vi "Drone Face Recognition.vi"() -> ()   [LabVIEW 2014]
doc: "This example shows how to use the Lucas Kanade Pyramid motion estimation VI to track features in a sequence of images in NI Vision. The VI reads the frames from an AVI file and tracks user specified features in the image from frame to frame."
uses:
  <vilib>/vision/NI_Vision_Development_Module.lvlib
panel:
  out "DroneGetVideoError":errorcluster
  out "Face Found":bool
  in  "Show Templates":bool=TRUE
  out "Preview":T1(plugin-control)
  in  "Lip Min Score":sgl=700.0
  in  "Nose Min Score":sgl=700.0
  in  "Eye Min Score":sgl=700.0
  out "Lips Template":T1(plugin-control)
  out "Nose Template":T1(plugin-control)
  out "Eye Template":T1(plugin-control)
  in  "Options":T2={"Level"=4, "maxiteration"=20, "windowsize"=20, "threshold"=1.0}
  in  "Stop":bool
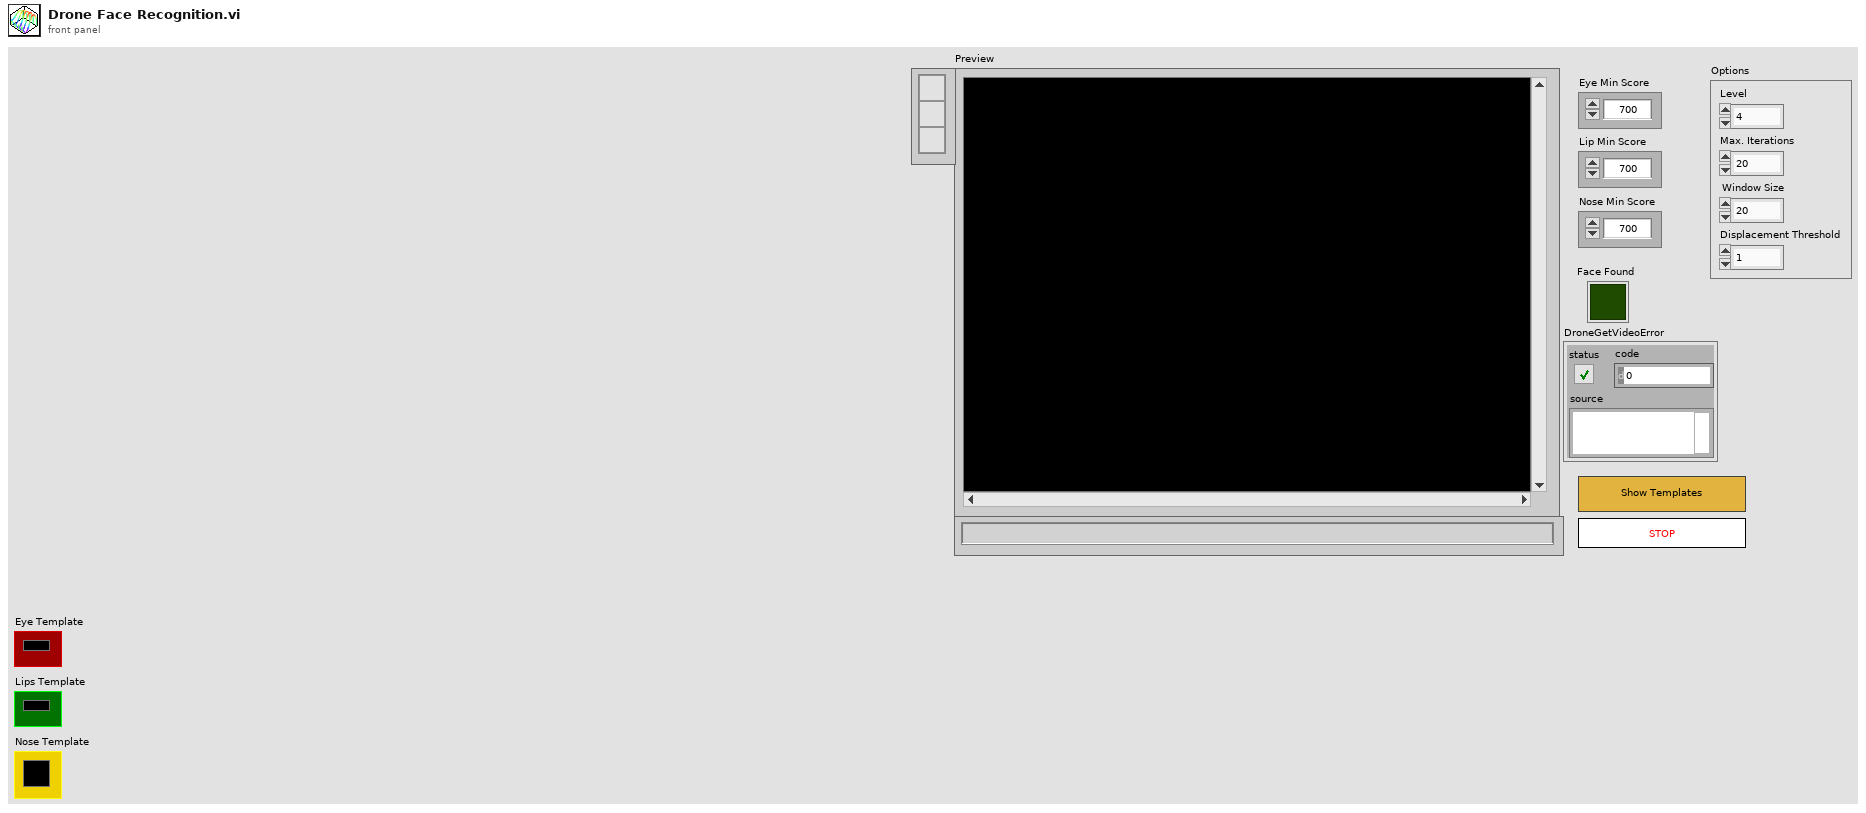
[diagram p1: front panel]
types:
  T1 = typedef "IMAQ Image.ctl" = refnum<image>
  T2 = cluster{"Level":i32, "maxiteration":i32, "windowsize":i32, "threshold":dbl}
  T3 = typedef "Image Type" = u32
  T4 = cluster{"Position":cluster{"x":sgl, "y":sgl}, "Angle":sgl, "Scale":sgl, "Score":sgl, "Bounding Box":cluster{"x":sgl, "y":sgl}[]}[]
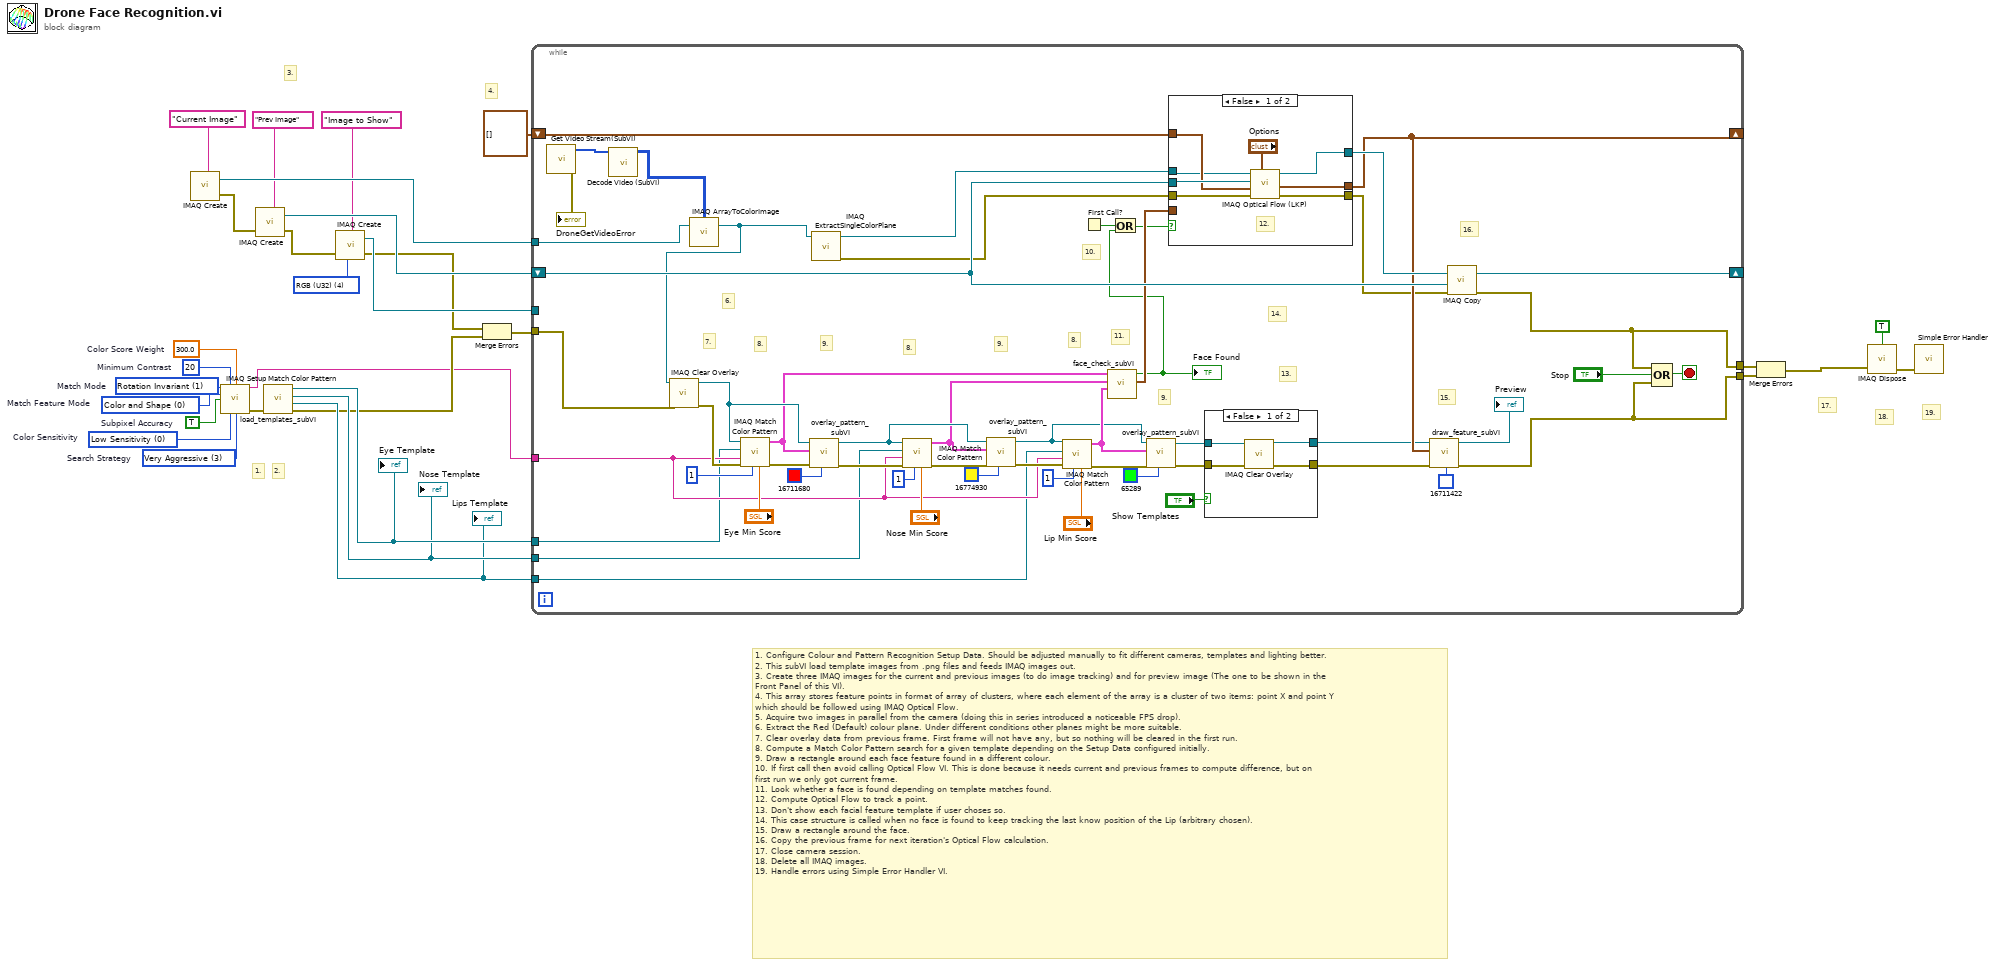
[diagram p0: block diagram]
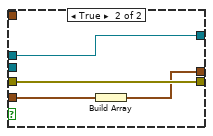
[diagram p3: hidden frame]
diagram:
  w15 = T3 4 items=["Grayscale (U8)", "Grayscale (I16)", "Grayscale (SGL)", "Complex (CSG)", "RGB (U32)", "HSL (U32)", "RGB (U64)", "Grayscale (U16)"] ("Image Type")
  w19 = TRUE  # Subpixel Accuracy
  w25 = u32 0 items=["Color and Shape", "Color", "Shape"]  # Match Feature Mode
  w24 = u32 3 items=["Conservative", "Balance", "Aggressive", "Very Aggressive"]  # Search Strategy
  w23 = 20  # Minimum Contrast
  w22 = sgl 300.0  # Color Score Weight
  w21 = u32 0 items=["Low Sensitivity", "Medium Sensitivity", "High Sensitivity"]  # Color Sensitivity
  w20 = u32 1 items=["Shift Invariant", "Rotation Invariant"]  # Match Mode
  # "1. Configure Colour and Pattern Recognition Setup Data. Should be adjusted manually to fit different cameras, templates and lighting better.\n2. This subVI load template images from .png files and feeds IMAQ images out.\n3. Create three IMAQ images for the current and previous images (to do image tracking) and for preview image (The one to be shown in the\nFront Panel of this VI).\n4. This array stores feature points in format of array of clusters, where each element of the array is a cluster of two items: point X and point Y \nwhich should be followed using IMAQ Optical Flow.\n5. Acquire two images in parallel from the camera (doing this in series introduced a noticeable FPS drop).\n6. Extract the Red (Default) colour plane. Under different conditions other planes might be more suitable.\n7. Clear overlay data from previous frame. First frame will not have any, but so nothing will be cleared in the first run.\n8. Compute a Match Color Pattern search for a given template depending on the Setup Data configured initially.\n9. Draw a rectangle around each face feature found in a different colour.\n10. If first call then avoid calling Optical Flow VI. This is done because it needs current and previous frames to compute difference, but on\nfirst run we only got current frame.\n11. Look whether a face is found depending on template matches found.\n12. Compute Optical Flow to track a point.\n13. Don't show each facial feature template if user choses so.\n14. This case structure is called when no face is found to keep tracking the last know position of the Lip (arbitrary chosen).\n15. Draw a rectangle around the face.\n16. Copy the previous frame for next iteration's Optical Flow calculation.\n17. Close camera session.\n18. Delete all IMAQ images.\n19. Handle errors using Simple Error Handler VI."
  # "19."
  # "17."
  # "4."
  # "3."
  # "3."
  # "3."
  # "2."
  # "1."
  # "18."
  n1 = call "IMAQ Create"("Image Name"="Current Image") -> ("New Image"=w29:T1, "error out"=w9:errorcluster)  [unwired: 3 in, 1 out]
  n2 = call "IMAQ Setup Match Color Pattern"("Match Mode"=w20, "Minimum Contrast"=w23, "Color Score Weight"=w22, "Match Feature Mode"=w25, "Subpixel Accuracy"=w19, "Color Sensitivity"=w21, "Search Strategy"=w24) -> ("Match Color Pattern Setup Data"=w4:string, "error out"=w18:errorcluster)  [unwired: 7 in]
  n3 = call "IMAQ Create"("Image Name"="Prev Image", "error in (no error)"=w9) -> ("New Image"=w26:T1, "error out"=w8:errorcluster)  [unwired: 2 in, 1 out]
  n4 = call "load_templates_subVI.vi"("error in (no error)"=w18) -> ("error out"=w6:errorcluster, "Lips Template"=w12:T1, "Nose Template"=w13:T1, "Eye Template"=w14:T1)  [unwired: 7 in]
  "Eye Template" <- w14
  "Nose Template" <- w13
  "Lips Template" <- w12
  n5 = call "IMAQ Create"("Image Name"="Image to Show", "Image Type"=w15, "error in (no error)"=w8) -> ("New Image"=w16:T1, "error out"=w7:errorcluster)  [unwired: 1 in, 1 out]
  n6 = Merge Errors(w7, w6) -> (w5:errorcluster)
  n7 = while {
    tunnel: w29 -> [w34]
    shift-right: [w83] -> _
    shift-left: w26 -> [w84]
    shift-right: [w51] -> _
    shift-left: cluster{"X":sgl, "Y":sgl}[] [] ("Feature Points Out") -> [w82]
    tunnel: w4 -> [w57]
    tunnel: w14 -> [w56]
    tunnel: w13 -> [w55]
    tunnel: w12 -> [w54]
    tunnel: w16 -> [_]
    tunnel: w5 -> [w36]
    tunnel: [w41] -> w3
    tunnel: [w40] -> w2
    stop <- w43 stop-if-true
    # "10."
    # "16."
    # "15."
    # "14."
    # "13."
    # "11."
    # "9."
    # "8."
    # "9."
    # "8."
    # "9."
    # "8."
    # "7."
    # "6."
    n8 = call "Get Video Stream(SubVI).vi"() -> ("error out"=→"DroneGetVideoError":errorcluster, "ImgData"=w35:u8[])  [unwired: 10 in]
    n9 = call "Decode Video (SubVI).vi"("ImgData"=w35) -> ("Array"=w32:u32[][])  [unwired: 9 in, 1 out]
    n10 = call "IMAQ ArrayToColorImage"("Image Pixels (U32)"=w32, "Image"=w34) -> ("Image Out"=w31:T1)  [unwired: 3 in, 1 out]
    n11 = call "IMAQ Clear Overlay"("error in (no error)"=w36, "Image"=w31) -> ("error out"=w78:errorcluster, "Image Out"=w64:T1)  [unwired: 8 in]
    n12 = call "IMAQ Match Color Pattern"("Minimum Match Score"="Eye Min Score", "Number of Matches Requested"=1, "error in (no error)"=w78, "Match Color Pattern Setup Data"=w57, "Template Image"=w56, "Image"=w64) -> ("error out"=w77:errorcluster, "Matches"=w61:T4)  [unwired: 3 in, 1 out]
    n13 = call "overlay_pattern_subVI.vi"("Color"=u32 16711680, "error in"=w77, "Matches"=w61, "Image"=w64) -> ("error out"=w74:errorcluster, "Image Out"=w71:T1)  [unwired: 6 in]
    n14 = call "IMAQ ExtractSingleColorPlane"("Image Src"=w31) -> ("error out"=w81:errorcluster, "Image Dst Out"=w80:T1)  [unwired: 9 in]
    n15 = call "IMAQ Match Color Pattern"("Minimum Match Score"="Nose Min Score", "Number of Matches Requested"=1, "error in (no error)"=w74, "Match Color Pattern Setup Data"=w57, "Template Image"=w55, "Image"=w71) -> ("error out"=w72:errorcluster, "Matches"=w60:T4)  [unwired: 3 in, 1 out]
    n16 = call "overlay_pattern_subVI.vi"("Color"=u32 16774930, "error in"=w72, "Matches"=w60, "Image"=w71) -> ("error out"=w70:errorcluster, "Image Out"=w58:T1)  [unwired: 6 in]
    n17 = call "IMAQ Match Color Pattern"("Minimum Match Score"="Lip Min Score", "Number of Matches Requested"=1, "error in (no error)"=w70, "Match Color Pattern Setup Data"=w57, "Template Image"=w54, "Image"=w58) -> ("error out"=w69:errorcluster, "Matches"=w59:T4)  [unwired: 3 in, 1 out]
    n18 = First Call?() -> (First Call?: T/F=w37:bool)
    n19 = call "face_check_subVI.vi"("Lips Match"=w59, "Nose Match"=w60, "Eye Match"=w61) -> ("Lip Position"=w53:cluster{"x":sgl, "y":sgl}, "Face Found"=w39:bool)  [unwired: 6 in, 1 out]
    "Face Found" <- w39
    n20 = Or(x=w37, y=w39) -> (x .or. y?=w38:bool)
    n21 = call "overlay_pattern_subVI.vi"("Color"=u32 65289, "error in"=w69, "Matches"=w59, "Image"=w58) -> ("error out"=w47:errorcluster, "Image Out"=w49:T1)  [unwired: 6 in]
    n22 = case shown="False" w38 {
      tunnel: w84 -> [w98 _]
      tunnel: w82 -> [w97 _]
      tunnel: [w96 w99] -> w51
      tunnel: w81 -> [w95 w102]
      tunnel: w80 -> [w91 w101]
      tunnel: [w93 w101] -> w79
      tunnel: [w92 w102] -> w44
      tunnel: w53 -> [_ w100]
      frame False {
        # "12."
        n23 = call "IMAQ Optical Flow (LKP)"("Options"="Options", "error in (no error)"=w95, "Feature Points In"=w97, "Previous Frame"=w98, "Current Frame"=w91) -> ("error out"=w92:errorcluster, "Feature Points Out"=w96:cluster{"X":sgl, "Y":sgl}[], "Current Frame Out (dup)"=w93:T1)  [unwired: 1 in, 3 out]
      }
      frame True {
        n24 = Build Array(w100) -> (w99:cluster{"x":sgl, "y":sgl}[])
      }
    }
    n25 = case shown="False" "Show Templates" {
      tunnel: w49 -> [w88 w90]
      tunnel: [w87 w90] -> w48
      tunnel: w47 -> [w86 w89]
      tunnel: [w85 w89] -> w45
      frame False {
        n26 = call "IMAQ Clear Overlay"("error in (no error)"=w86, "Image"=w88) -> ("error out"=w85:errorcluster, "Image Out"=w87:T1)  [unwired: 8 in]
      }
      frame True {
      }
    }
    n27 = call "draw_feature_subVI.vi"("Color"=u32 16711422, "Error In"=w45, "Feature Ponts"=w51, "Image"=w48) -> ("Error Out"=w40:errorcluster, "Image Out"=→"Preview":T1)  [unwired: 6 out]
    n28 = call "IMAQ Copy"("error in (no error)"=w44, "Image Dst"=w84, "Image Src"=w79) -> ("error out"=w41:errorcluster, "Image Dst Out"=w83:T1)  [unwired: 3 out]
    n29 = Compound Arithmetic op=OR(w41, "Stop", w40) -> (w43:bool)
  }
  n30 = Merge Errors(w3, w2) -> (w1:errorcluster)
  n31 = call "IMAQ Dispose"("All Images? (No)"=TRUE, "error in (no error)"=w1) -> ("error out"=w11:errorcluster)  [unwired: 1 in, 3 out]
  n32 = call <vilib>:"Simple Error Handler.vi"("error in (no error)"=w11) -> ()  [unwired: 1 in, 8 out]
